vi "Build Picture.vi"(11 "data string":string) -> (3 "Last Image":string)   [LabVIEW 2019]
panel:
  out "length 2":i32
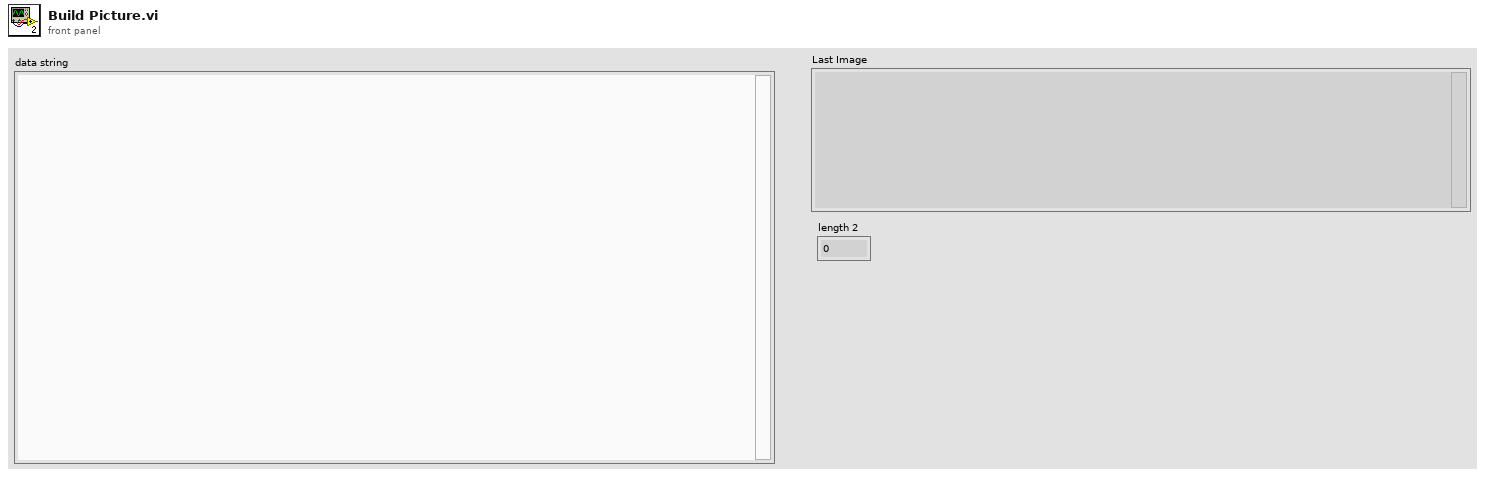
[diagram p1: front panel]
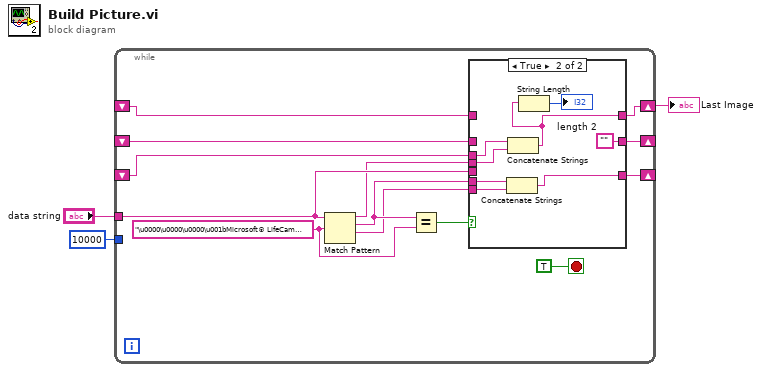
[diagram p0: block diagram]
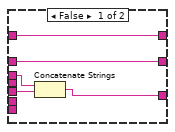
[diagram p2: hidden frame]
diagram:
  n1 = while {
    tunnel: 10000 ("length (rest)") -> [_]
    shift-right: [w15] -> _
    shift-left: _ -> [w14]
    shift-right: [w9] -> _
    shift-left: _ -> [w8]
    tunnel: "data string" -> [w16]
    shift-right: [w5] -> w1
    shift-left: _ -> [w4]
    stop <- TRUE stop-if-true
    w10 = "\u0000\u0000\u0000\u001bMicrosoft® LifeCam HD-3000" ("regular expression")
    n2 = Match Pattern(string=w16, regular expression=w10) -> (before substring=w12:string, match substring=w11:string, after substring=w7:string)  [unwired: 1 in, 1 out]
    n3 = Equal?(x=w11, y=w10) -> (x = y?=w13:bool)
    n4 = case shown="True" w13 {
      tunnel: [w18 ""] -> w15
      tunnel: w14 -> [w18 _]
      tunnel: w12 -> [_ w29]
      tunnel: w11 -> [_ w28]
      tunnel: w7 -> [_ w27]
      tunnel: [w19 w26] -> w9
      tunnel: w16 -> [w21 _]
      tunnel: w8 -> [w20 w25]
      tunnel: [w17 w22] -> w5
      tunnel: w4 -> [w17 _]
      frame False {
        n5 = Concatenate Strings(w20, w21) -> (w19:string)
      }
      frame True {
        n6 = Concatenate Strings(w28, w27) -> (w26:string)
        n7 = Concatenate Strings(w25, w29) -> (w22:string)
        n8 = String Length(string=w22) -> (length=→"length 2":i32)
      }
    }
  }
  "Last Image" <- w1
